vi "Frame_CRC_check.vi"(8 "error in (no error)":errorcluster, 11 "ISO 14443 A DOWN in":refnum<class "ISO 14443 A DOWN.lvclass">) -> (0 "error out":errorcluster, 3 "ISO 14443 A DOWN out":refnum<class "ISO 14443 A DOWN.lvclass">)   [LabVIEW 2019, in "ISO 14443 A DOWN.lvclass"]
uses:
  ISO 14443 A DOWN.lvclass
  ISO 14443 A DOWN.lvclass/ISO 14443 A DOWN.ctl
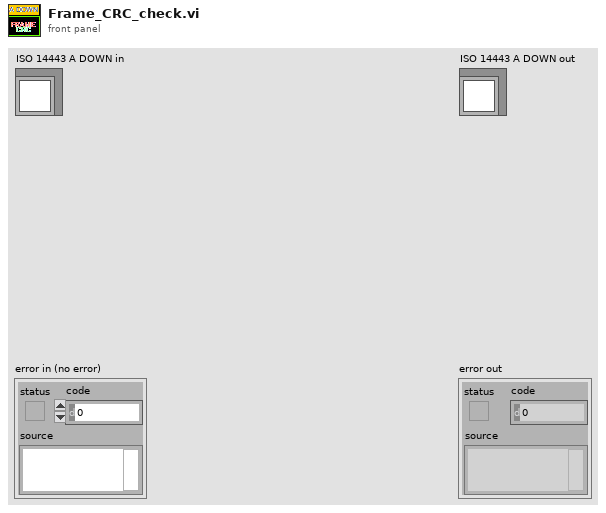
[diagram p1: front panel]
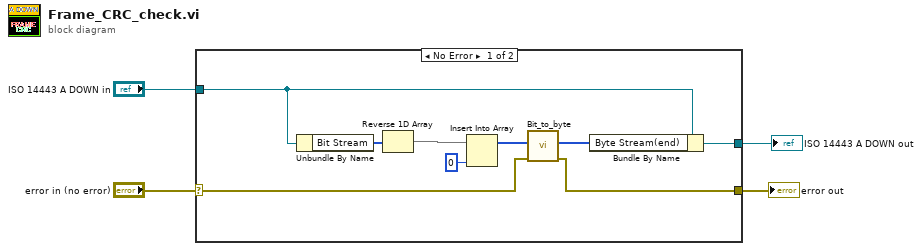
[diagram p0: block diagram]
diagram:
  n1 = case shown="No Error" "error in (no error)" {
    selector: "error in (no error)" -> [w9 w14]
    tunnel: [w8 w14] -> w3
    tunnel: "ISO 14443 A DOWN in" -> [w12 w15]
    tunnel: [w11 w15] -> w1
    frame No Error {
      n2 = Unbundle By Name(w12) -> ("Bit Stream"=w7:u8[])
      n3 = Reverse 1D Array(array=w7) -> (reversed array=w6:u8[])
      n4 = Insert Into Array(array=w6, new element=u8 0 ("new element/subarray")) -> (w13:u8[])  [unwired: 1 in]
      n5 = call "Bit_to_byte.vi"("Error In"=w9, "Array of bit"=w13) -> ("Error Out"=w8:errorcluster, "Array of byte"=w10:u8[])  [unwired: 7 in, 1 out]
      n6 = Bundle By Name(cluster=w12, "Byte Stream(end)"=w10) -> (w11:refnum<class "ISO 14443 A DOWN.lvclass">)
    }
    frame Error {
    }
  }
  "error out" <- w3
  "ISO 14443 A DOWN out" <- w1
